vi "remove tag from table.vi"(9 "index":i32, 10 "data type":T1, 11 "data table in":T2) -> (3 "data table out":T2)   [LabVIEW 2013, in "data bus values.lvlib"]
doc: "Removes a specified tag, by type and index, from the data table."
uses:
  data bus values.lvlib
  data table.ctl
  tag/Data Type.ctl
  tag/data bus tag description.lvclass
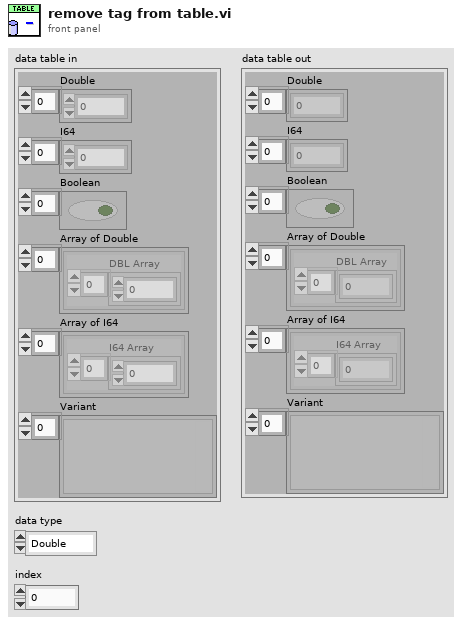
[diagram p1: front panel]
types:
  T1 = typedef "data bus tag description.lvclass/Data Type.ctl" = enum16{"Double", "I64", "Boolean", "Array of Double", "Array of I64", "Variant"}
  T2 = typedef "data bus values.lvlib/data table.ctl" = cluster{"Double":dbl[], "I64":i64[], "Boolean":bool[], "Array of Double":cluster{"DBL Array":dbl[]}[], "Array of I64":cluster{"I64 Array":i64[]}[], "Variant":variant[]}
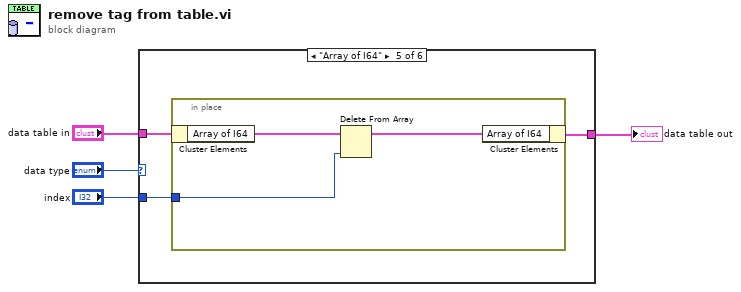
[diagram p0: block diagram]
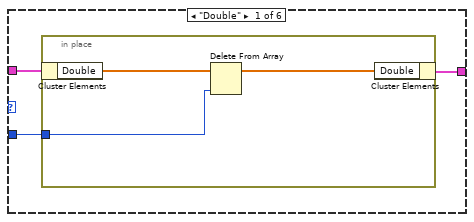
[diagram p2: hidden frame]
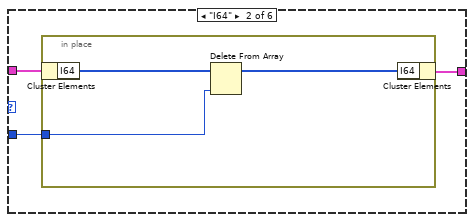
[diagram p3: hidden frame]
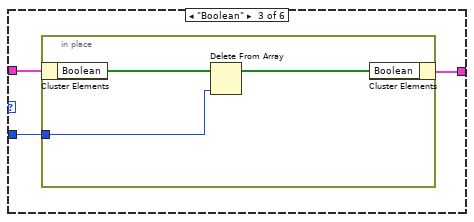
[diagram p4: hidden frame]
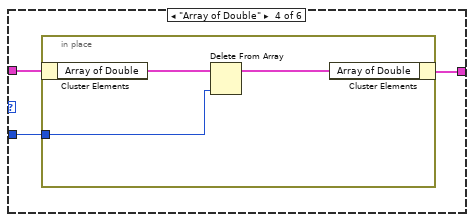
[diagram p5: hidden frame]
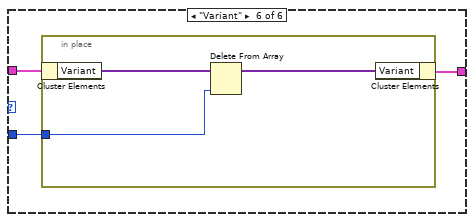
[diagram p6: hidden frame]
diagram:
  n1 = case shown="\"Array of I64\"" "data type" {
    tunnel: "data table in" -> [w7 w13 w19 w25 w31 w37]
    tunnel: [w6 w12 w18 w24 w30 w36] -> w3
    tunnel: "index" -> [w5 w11 w17 w23 w29 w35]
    frame "Double" {
      n2 = in-place {
        in-place-border: w5 -> [w8]
        n3 = in-place-cluster #1(w7) -> ("Double"=w10:dbl[])
        n4 = Delete From Array(array=w10, index=w8) -> (array with subset deleted=w9:dbl[])  [unwired: 1 in, 1 out]
        n5 = in-place-cluster #1("Double"=w9) -> (w6:T2)
      }
    }
    frame "I64" {
      n6 = in-place {
        in-place-border: w11 -> [w14]
        n7 = in-place-cluster #2(w13) -> ("I64"=w16:i64[])
        n8 = Delete From Array(array=w16, index=w14) -> (array with subset deleted=w15:i64[])  [unwired: 1 in, 1 out]
        n9 = in-place-cluster #2("I64"=w15) -> (w12:T2)
      }
    }
    frame "Boolean" {
      n10 = in-place {
        in-place-border: w17 -> [w20]
        n11 = in-place-cluster #3(w19) -> ("Boolean"=w22:bool[])
        n12 = Delete From Array(array=w22, index=w20) -> (array with subset deleted=w21:bool[])  [unwired: 1 in, 1 out]
        n13 = in-place-cluster #3("Boolean"=w21) -> (w18:T2)
      }
    }
    frame "Array of Double" {
      n14 = in-place {
        in-place-border: w23 -> [w26]
        n15 = in-place-cluster #4(w25) -> ("Array of Double"=w28:cluster{"DBL Array":dbl[]}[])
        n16 = Delete From Array(array=w28, index=w26) -> (array with subset deleted=w27:cluster{"DBL Array":dbl[]}[])  [unwired: 1 in, 1 out]
        n17 = in-place-cluster #4("Array of Double"=w27) -> (w24:T2)
      }
    }
    frame "Array of I64" {
      n18 = in-place {
        in-place-border: w29 -> [w32]
        n19 = in-place-cluster #5(w31) -> ("Array of I64"=w34:cluster{"I64 Array":i64[]}[])
        n20 = Delete From Array(array=w34, index=w32) -> (array with subset deleted=w33:cluster{"I64 Array":i64[]}[])  [unwired: 1 in, 1 out]
        n21 = in-place-cluster #5("Array of I64"=w33) -> (w30:T2)
      }
    }
    frame "Variant" {
      n22 = in-place {
        in-place-border: w35 -> [w38]
        n23 = in-place-cluster #6(w37) -> ("Variant"=w40:variant[])
        n24 = Delete From Array(array=w40, index=w38) -> (array with subset deleted=w39:variant[])  [unwired: 1 in, 1 out]
        n25 = in-place-cluster #6("Variant"=w39) -> (w36:T2)
      }
    }
  }
  "data table out" <- w3
